vi "Transaction.vi"(0 "VisaCluster":T1, 5 "Command":string, 7 "Time (150) ms":u32=150, 9 "Read Only? (False)":bool, 11 "error in (no error)":errorcluster) -> (4 "VisaCluster":T1, 6 "Answer":string, 10 "bytes read":u32, 15 "error out":errorcluster)   [LabVIEW 2014, in "FH 55.lvlib"]
doc: "Communication with instrument. Send commands and read answer."
uses:
  FH 55.lvlib
  TypeDef/VisaCluster.ctl
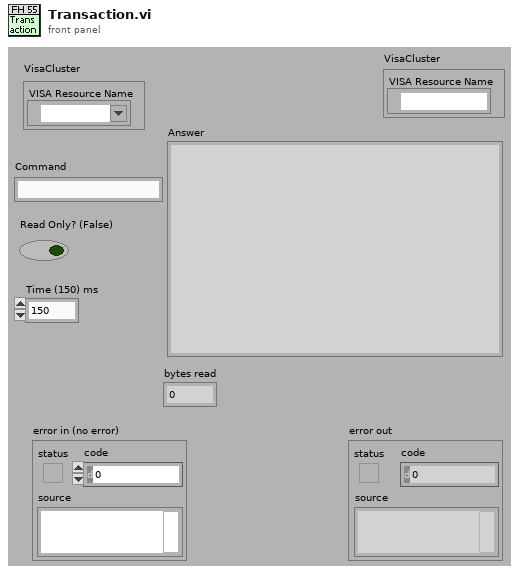
[diagram p1: front panel]
types:
  T1 = typedef "FH 55.lvlib/VisaCluster.ctl" = cluster{"VISA Resource Name":refnum<visa-resource-name>}
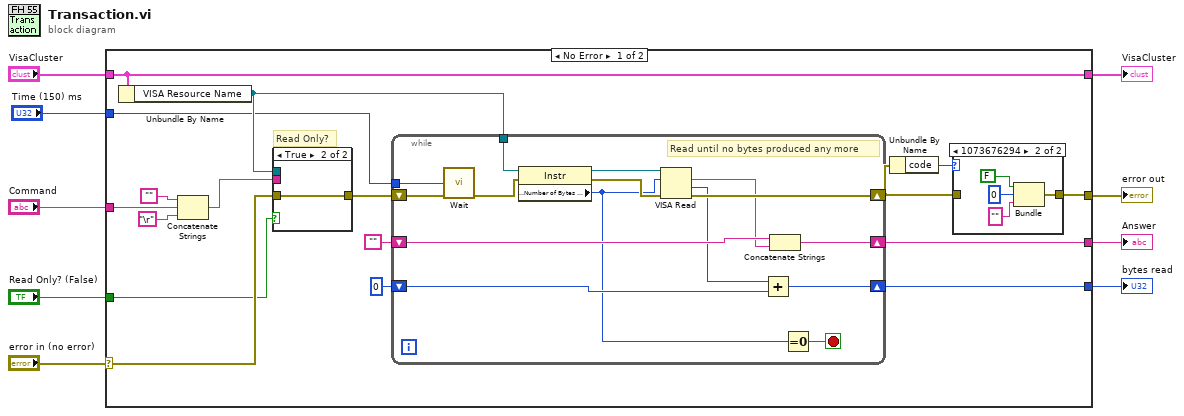
[diagram p0: block diagram]
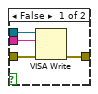
[diagram p3: hidden frame]
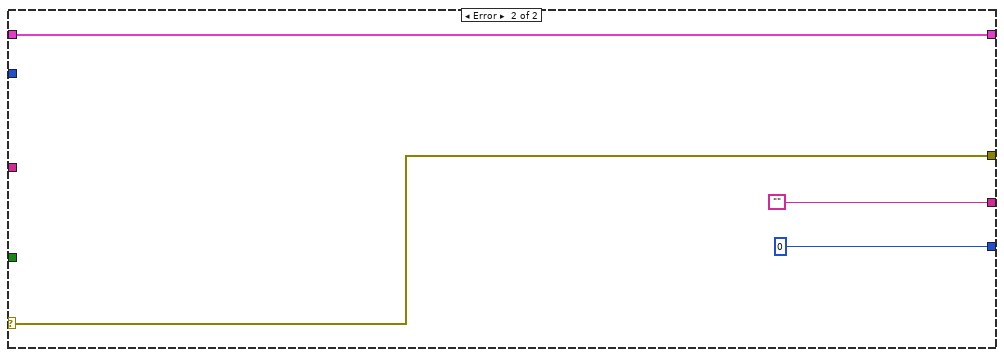
[diagram p4: hidden frame]
diagram:
  n1 = case shown="No Error" "error in (no error)" {
    selector: "error in (no error)" -> [w26 w55]
    tunnel: [w13 w55] -> w6
    tunnel: "VisaCluster" -> [w24 w54]
    tunnel: [w24 w54] -> w2
    tunnel: "Command" -> [w22 _]
    tunnel: [w25 "" ("read buffer")] -> w5
    tunnel: [w17 u32 0] -> w4
    tunnel: "Read Only? (False)" -> [w16 _]
    tunnel: "Time (150) ms" -> [w10 _]
    frame No Error {
      # "Read Only?"
      n2 = Unbundle By Name(w24) -> ("VISA Resource Name"=w23:refnum<visa-resource-name>)
      n3 = Concatenate Strings("", w22, "\r") -> (w21:string)
      n4 = case shown="True" w16 {
        tunnel: w26 -> [w35 w36]
        tunnel: w23 -> [w34 _]
        tunnel: w21 -> [w33 _]
        tunnel: [w32 w36] -> w20
        frame False {
          n5 = VISA Write(VISA resource name=w34, write buffer=w33, error in (no error)=w35) -> (error out=w32:errorcluster)  [unwired: 2 out]
        }
        frame True {
        }
      }
      n6 = while {
        tunnel: w23 -> [w48]
        shift-right: [w45] -> w25
        shift-left: "" -> [w47]
        shift-right: [w42] -> w17
        shift-left: u32 0 -> [w44]
        shift-right: [w51] -> w14
        shift-left: w20 -> [w40]
        tunnel: w10 -> [w37]
        stop <- w38 stop-if-true
        # "Read until no bytes produced any more"
        n7 = call "Wait.vi"("milliseconds to wait"=w37, "error in (no error)"=w40) -> ("error out"=w39:errorcluster)  [unwired: 13 in]
        n8 = property class="Instr"(reference=w48, error in=w39) -> (reference out=w50:refnum<visa-resource-name>, error out=w49:errorcluster, "Serial Settings:Number of Bytes at Serial Port"=w41:u32)
        n9 = VISA Read(VISA resource name=w50, byte count=w41, error in (no error)=w49) -> (read buffer=w46:string, return count=w43:u32, error out=w51:errorcluster)  [unwired: 1 out]
        n10 = Add(x=w43, y=w44) -> (x+y=w42:u32)
        n11 = Concatenate Strings(w47, w46) -> (w45:string)
        n12 = Equal To 0?(x=w41) -> (x = 0?=w38:bool)
      }
      n13 = Unbundle By Name(w14) -> ("code"=w15:i32)
      n14 = case shown="1073676294" w15 {
        tunnel: [w27 w28] -> w13
        tunnel: w14 -> [w27 _]
        frame 0, Default {
        }
        frame 1073676294 {
          n15 = Bundle(FALSE, 0, "") -> (w28:errorcluster)  [unwired: 1 in]
        }
      }
    }
    frame Error {
    }
  }
  "error out" <- w6
  "Answer" <- w5
  "bytes read" <- w4
  "VisaCluster" <- w2
